vi "AddVIDocument.vi"   [LabVIEW 2011]
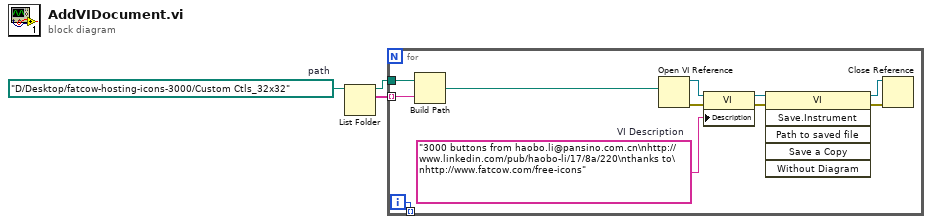
[diagram p0: block diagram]
diagram:
  w3 = path "D:/Desktop/fatcow-hosting-icons-3000/Custom Ctls_32x32"  # path
  n1 = List Folder(path=w3) -> (path out=w2:path, filenames=w1:string[])  [unwired: 3 in, 2 out]
  n2 = for {
    tunnel: w2 -> [w14]
    tunnel: w1 -> [w13] mode=indexing
    tunnel: [w4] -> _ mode=indexing
    i -> [w4]
    w10 = "3000 buttons from haobo.li@pansino.com.cn\nhttp://www.linkedin.com/pub/haobo-li/17/8a/220\nthanks to\nhttp://www.fatcow.com/free-icons"  # VI Description
    n3 = Build Path(base path=w14, name or relative path=w13) -> (appended path=w12:path)
    n4 = Open VI Reference(vi path=w12) -> (vi reference=w11:refnum<vi>, error out=w7:errorcluster)  [unwired: 5 in]
    n5 = property class="VI"(reference=w11, error in=w7, "Description"=w10) -> (reference out=w9:refnum<vi>, error out=w6:errorcluster)
    n6 = invoke class="VI" method="Save.Instrument"(reference=w9, error in=w6) -> (reference out=w8:refnum<vi>, error out=w5:errorcluster)  [unwired: 4 in, 4 out]
    n7 = Close Reference(reference=w8, error in (no error)=w5) -> ()  [unwired: 1 out]
  }
